vi "加标回收数据处理整合 (子VI).vi"(11 "枚举":enum16{"实时数据排序", "小时数据排序"}(ring)) -> (3 "已排序的数组":string[](array[string]))   [LabVIEW 2016, in "数据传输系统-02.lvlib"]
uses:
  <userlib>/_OpenG.lib/array/array.llb/Remove Duplicates from 1D Array (String)__ogtk.vi
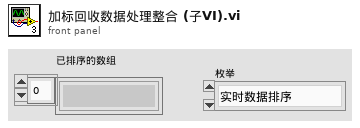
[diagram p1: front panel]
types:
  T1 = cluster{"PH":string[][], "CODCr":string[][], "氨氮":string[][], "CODMn":string[][], "总氮":string[][], "总磷":string[][], "电导率":string[][], "水温":string[][], "DO":string[][], "浊度":string[][], "叶绿素":string[][], "藻密度":string[][], "铜":string[][], "盐度":string[][], "水位":string[][], "流速":string[][], "瞬时流量":string[][], "累积流量":string[][], "亚硝酸盐":string[][], "硫化物":string[][], "ORP":string[][], "铅":string[][], "镉":string[][], "锌":string[][], "镍":string[][], "锰":string[][], "汞":string[][], "气温":string[][], "气压":string[][], "风速":string[][], "风向":string[][], "盐度 2":string[][], "磷酸盐":string[][], "硝氮":string[][], "氟化物":string[][], "挥发酚":string[][], "氯化物":string[][]}
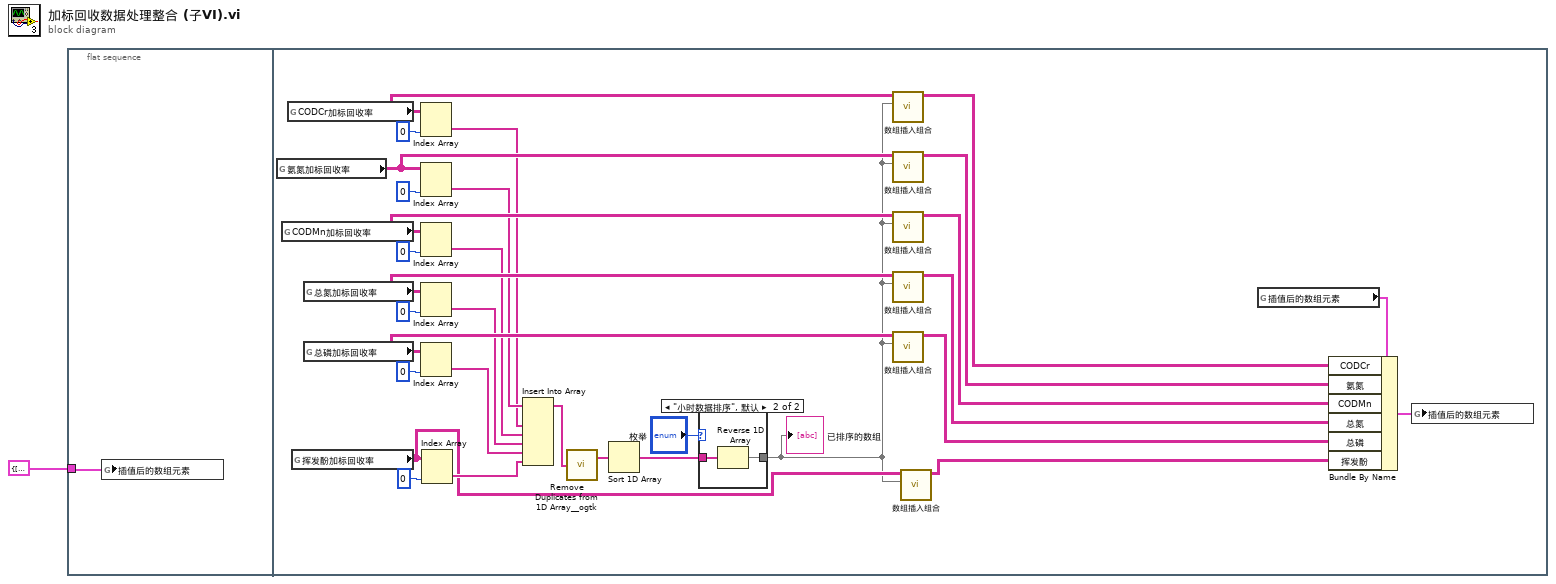
[diagram p0: block diagram]
diagram:
  n1 = flat-sequence {
    tunnel: T1 {"PH"=[], "CODCr"=[], "氨氮"=[], "CODMn"=[], "总氮"=[], "总磷"=[], "电导率"=[], "水温"=[], "DO"=[], "浊度"=[], "叶绿素"=[], "藻密度"=[], "铜"=[], "盐度"=[], "水位"=[], "流速"=[], "瞬时流量"=[], "累积流量"=[], "亚硝酸盐"=[], "硫化物"=[], "ORP"=[], "铅"=[], "镉"=[], "锌"=[], "镍"=[], "锰"=[], "汞"=[], "气温"=[], "气压"=[], "风速"=[], "风向"=[], "盐度 2"=[], "磷酸盐"=[], "硝氮"=[], "氟化物"=[], "挥发酚"=[], "氯化物"=[]} ("插值后的数组元素") -> [w2]
    frame #0 {
      n2 = global write "插值后的新数组.vi" "插值后的数组元素"(w2) -> ()
    }
    frame #1 {
      n3 = global read "全局 所有参数.vi" "氨氮加标回收率"() -> (w15:string[][])
      n4 = global read "全局 所有参数.vi" "CODMn加标回收率"() -> (w26:string[][])
      n5 = global read "全局 所有参数.vi" "CODCr加标回收率"() -> (w25:string[][])
      n6 = global read "全局 所有参数.vi" "挥发酚加标回收率"() -> (w5:string[][])
      n7 = global read "全局 所有参数.vi" "总氮加标回收率"() -> (w27:string[][])
      n8 = global read "全局 所有参数.vi" "总磷加标回收率"() -> (w28:string[][])
      n9 = Index Array(array=w25, index (col)=0 ("索引 (行)")) -> (element=w13:string[])  [unwired: 1 in]
      n10 = Index Array(array=w15, index (col)=0 ("索引 (行)")) -> (element=w14:string[])  [unwired: 1 in]
      n11 = Index Array(array=w26, index (col)=0 ("索引 (行)")) -> (element=w12:string[])  [unwired: 1 in]
      n12 = Index Array(array=w27, index (col)=0 ("索引 (行)")) -> (element=w11:string[])  [unwired: 1 in]
      n13 = Index Array(array=w28, index (col)=0 ("索引 (行)")) -> (element=w10:string[])  [unwired: 1 in]
      n14 = Index Array(array=w5, index (col)=0 ("索引 (行)")) -> (element=w6:string[])  [unwired: 1 in]
      n15 = Insert Into Array(array=w14, new element #1=w13, new element #2=w12, new element #3=w11, new element #4=w10, new element #5=w6) -> (w24:string[])  [unwired: 1 in]
      n16 = call-poly <userlib>:"Remove Duplicates from 1D Array__ogtk.vi"("Input Array"=w24) -> ("Output Array"=w23:string[])  [unwired: 1 out]
      n17 = Sort 1D Array(array=w23) -> (sorted array=w16:string[])
      n18 = case shown="\"小时数据排序\", 默认" "枚举" {
        tunnel: w16 -> [w34 w36]
        tunnel: [w34 w35] -> w4
        frame "实时数据排序" {
        }
        frame "小时数据排序", Default {
          n19 = Reverse 1D Array(array=w36) -> (reversed array=w35:string[])
        }
      }
      "已排序的数组" <- w4
      n20 = call "数组插入组合.vi"("排序后的一维数组"=w4, "输入数组"=w25) -> ("输出结果"=w29:string[][])  [unwired: 9 in]
      n21 = call "数组插入组合.vi"("排序后的一维数组"=w4, "输入数组"=w15) -> ("输出结果"=w30:string[][])  [unwired: 9 in]
      n22 = call "数组插入组合.vi"("排序后的一维数组"=w4, "输入数组"=w26) -> ("输出结果"=w31:string[][])  [unwired: 9 in]
      n23 = call "数组插入组合.vi"("排序后的一维数组"=w4, "输入数组"=w27) -> ("输出结果"=w32:string[][])  [unwired: 9 in]
      n24 = call "数组插入组合.vi"("排序后的一维数组"=w4, "输入数组"=w28) -> ("输出结果"=w33:string[][])  [unwired: 9 in]
      n25 = call "数组插入组合.vi"("排序后的一维数组"=w4, "输入数组"=w5) -> ("输出结果"=w3:string[][])  [unwired: 9 in]
      n26 = global read "插值后的新数组.vi" "插值后的数组元素"() -> (w9:T1)
      n27 = Bundle By Name(cluster=w9, "CODCr"=w29, "氨氮"=w30, "CODMn"=w31, "总氮"=w32, "总磷"=w33, "挥发酚"=w3) -> (w8:T1)
      n28 = global write "插值后的新数组.vi" "插值后的数组元素"(w8) -> ()
    }
  }
